vi "Write Job Name.vi"(8 "error in (no error)":errorcluster, 10 "Job Name":string, 11 "Cron.Jenkins in":refnum<class "Cron.Jenkins.lvclass">) -> (0 "error out":errorcluster, 3 "Cron.Jenkins out":refnum<class "Cron.Jenkins.lvclass">)   [LabVIEW 2013, in "openCron.lvlib" / "Cron.Jenkins.lvclass"]
uses:
  Cron.Jenkins.lvclass
  Cron.Jenkins.lvclass/Cron.Jenkins.ctl
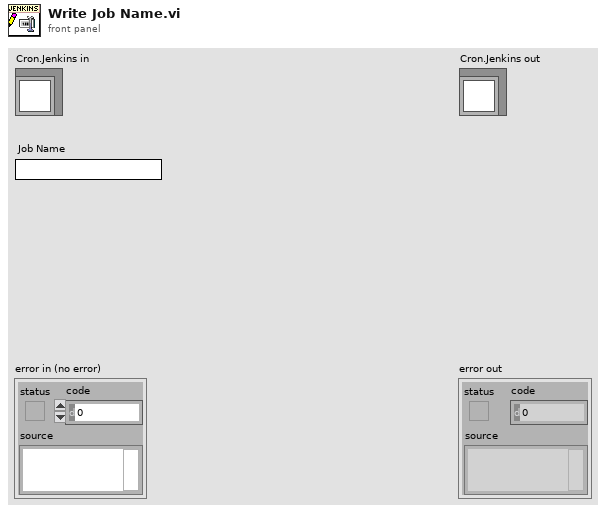
[diagram p1: front panel]
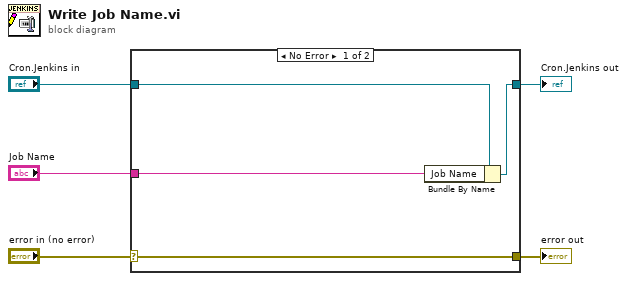
[diagram p0: block diagram]
diagram:
  n1 = case shown="No Error" "error in (no error)" {
    selector: "error in (no error)" -> [w9 w10]
    tunnel: [w9 w10] -> w4
    tunnel: [w7 w11] -> w2
    tunnel: "Cron.Jenkins in" -> [w8 w11]
    tunnel: "Job Name" -> [w6 _]
    frame No Error {
      n2 = Bundle By Name(cluster=w8, "Job Name"=w6) -> (w7:refnum<class "Cron.Jenkins.lvclass">)
    }
    frame Error {
    }
  }
  "error out" <- w4
  "Cron.Jenkins out" <- w2
